vi "Status.vi"(8 "error in (no error)":errorcluster, 11 "Queue in":refnum<queue>) -> (0 "error out":errorcluster, 1 "Running":bool[](array[boolean]), 2 "Timer Messages":string[](array[string]), 3 "Queue out":refnum<queue>, 4 "Delay (ms)":i32[](array[numeric]), 5 "Last Ticks (ms)":u32[](array[numeric]))   [LabVIEW 2018, in "QueueTimer.lvlib"]
doc: "Return the status and last enqueued ms tick counts of all queue timers associated with the <b>Queue</b> reference."
uses:
  QueueTimer.lvlib
  <vilib>/ErrorRing/Error Ring.xnode
  <vilib>/Utility/error.llb/Error Cluster From Error Code.vi
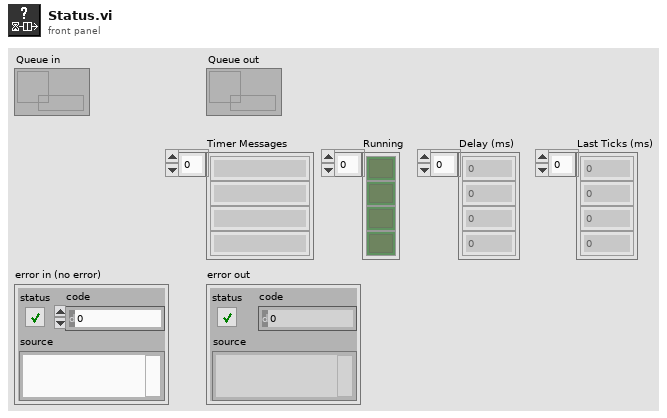
[diagram p1: front panel]
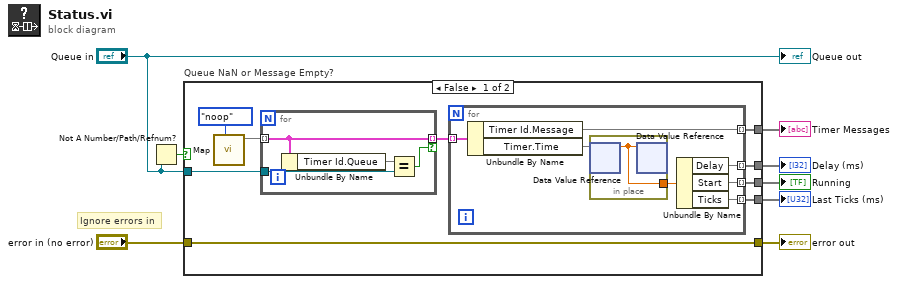
[diagram p0: block diagram]
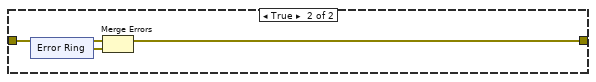
[diagram p2: hidden frame]
diagram:
  # "Ignore errors in"
  n1 = Not A Number/Path/Refnum?(number/path/refnum="Queue in") -> (NaN/Path/Refnum?=w6:bool)
  n2 = case "Queue NaN or Message Empty?" shown="False" w6 {
    tunnel: "Queue in" -> [w16 _]
    tunnel: "error in (no error)" -> [w14 w32]
    tunnel: [w14 w31] -> w7
    tunnel: [w12 _] -> w5
    tunnel: [w11 _] -> w4
    tunnel: [w10 _] -> w3
    tunnel: [w9 _] -> w2
    frame False {
      n3 = call "Map.vi"("Action"=enum8{"noop", "get", "set", "pop"}."noop") -> (3:w15)  [unwired: 8 in, 2 out]
      n4 = for {
        tunnel: w16 -> [w29]
        tunnel: w15 -> [w27] mode=indexing
        tunnel: [w27] -> w13 mode=indexing if=w26
        n5 = Unbundle By Name(w27) -> ("Timer Id.Queue"=w28)
        n6 = Equal?(x=w28, y=w29) -> (x = y?=w26:bool)
      }
      n7 = for {
        tunnel: w13 -> [w24] mode=indexing
        tunnel: [w23] -> w12 mode=indexing
        tunnel: [w20] -> w11 mode=indexing
        tunnel: [w19] -> w10 mode=indexing
        tunnel: [w18] -> w9 mode=indexing
        n8 = Unbundle By Name(w24) -> ("Timer Id.Message"=w23, "Timer.Time"=w22)
        n9 = in-place {
          in-place-border: [w25] -> w21
          n10 = in-place-dvr #1(w22) -> (w25:dbl)  [unwired: 1 out]
          n11 = in-place-dvr #1(w25) -> ()  [unwired: 2 out]
        }
        n12 = Unbundle By Name(w21) -> ("Delay"=w20, "Start"=w19, "Ticks"=w18)
      }
    }
    frame True {
      n13 = xnode "Error Ring"() -> ("error out"=w30:errorcluster)
      n14 = Merge Errors(w32, w30) -> (w31:errorcluster)
    }
  }
  "error out" <- w7
  "Timer Messages" <- w5
  "Delay (ms)" <- w4
  "Running" <- w3
  "Last Ticks (ms)" <- w2
  "Queue out" <- "Queue in"
